vi "Copy Builds NI VeriStand dir.vi"(8 "error in (no error)":errorcluster, 9 "Custom Device Name":string="TimingDRV", 10 "VS Common Directory":string="Timing and Sync", 11 "CD Build Tools in":refnum<class "Project Build Tools.lvclass">) -> (0 "error out":errorcluster, 3 "CD Build Tools out":refnum<class "Project Build Tools.lvclass">)   [LabVIEW 2019, in "Project Build Tools.lvclass"]
doc: "This VI is called after each run of a build specification. The VI will copy the generated LLB (Engine or System Explorer) into the VeriStand Custom Device folder (...\\Documents\\National Instruments\\NI VeriStand 2013...)."
uses:
  Project Build Tools.lvclass
  <vilib>/Utility/sysdir.llb/System Directory Type.ctl
  Project Build Tools.lvclass/Project Build Tools.ctl
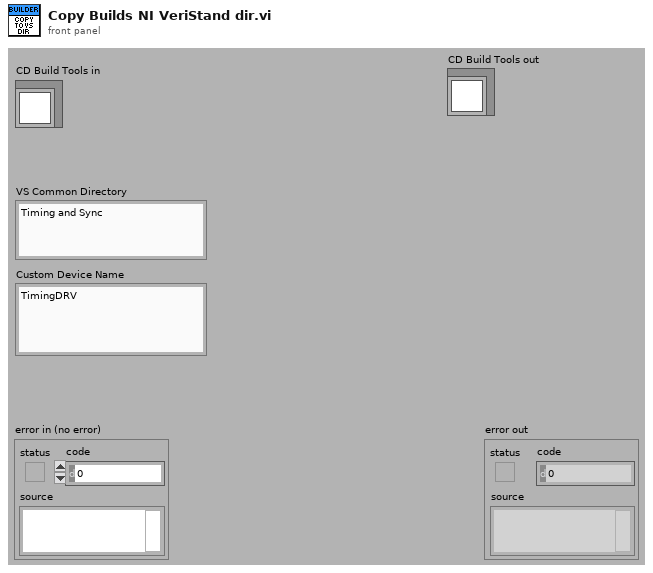
[diagram p1: front panel]
types:
  T1 = typedef "System Directory Type.ctl" = i32
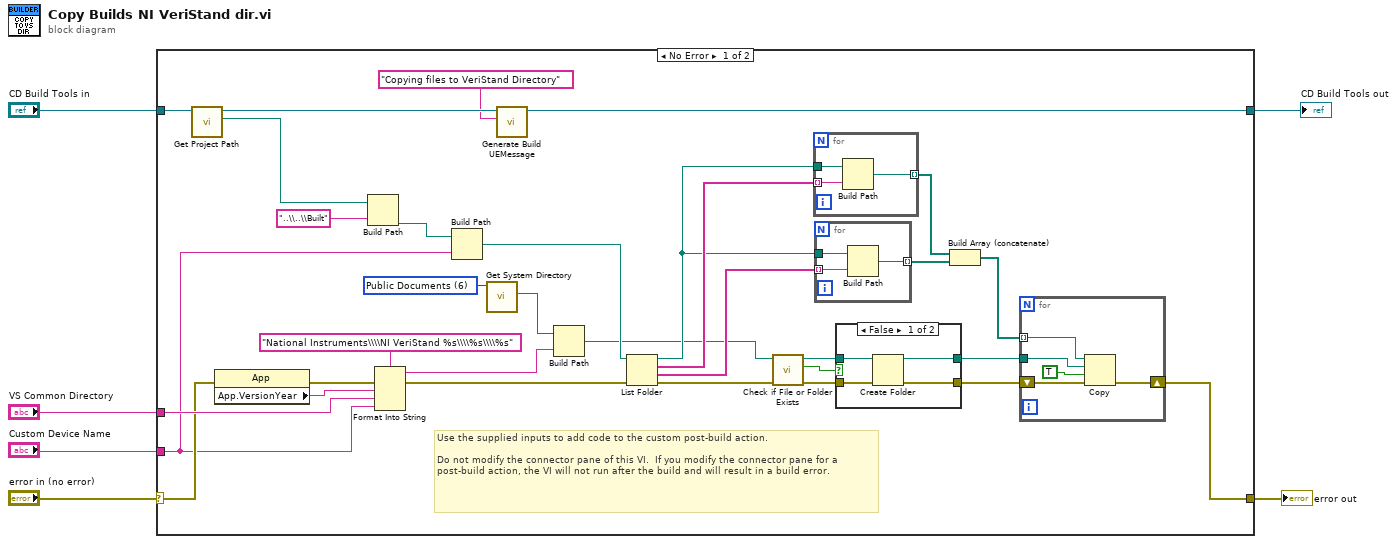
[diagram p0: block diagram]
diagram:
  n1 = case shown="No Error" "error in (no error)" {
    selector: "error in (no error)" -> [w17 w57]
    tunnel: [w20 w57] -> w5
    tunnel: "VS Common Directory" -> [w18 _]
    tunnel: "Custom Device Name" -> [w15 _]
    tunnel: "CD Build Tools in" -> [w11 w56]
    tunnel: [w7 w56] -> w1
    frame No Error {
      w24 = T1 6 items=["User Home"=0, "User Desktop"=1, "User Documents"=2, "User Application Data"=3, "User Preferences"=4, "User Temporary"=5, "Public Documents"=6, "Public Application Data"=7, "Public Preferences"=8, "Public Cache"=13, "System Core Libraries"=9, "System Installed Libraries"=10, "Application Files"=11, "Boot Volume Root"=12] ("system directory type")
      # "Use the supplied inputs to add code to the custom post-build action.\n\nDo not modify the connector pane of this VI.  If you modify the connector pane for a post-build action, the VI will not run after the build and will result in a build error."
      n2 = call "Get Project Path.vi"("CD Build Tools in"=w11) -> ("Project Path"=w10:path, "CD Build Tools out"=w9:refnum<class "Project Build Tools.lvclass">)  [unwired: 9 in]
      n3 = property class="App"(error in=w17) -> (error out=w23:errorcluster, "App.VersionYear"=w22:string)  [unwired: 1 in, 1 out]
      n4 = Build Path(base path=w10, name or relative path="..\\..\\Built") -> (appended path=w27:path)
      n5 = Format Into String(format string="National Instruments\\\\NI VeriStand %s\\\\%s\\\\%s" ("name or relative path"), error in=w23, w22, w18, w15) -> (resulting string=w26:string, error out=w16:errorcluster)  [unwired: 1 in]
      n6 = Build Path(base path=w27, name or relative path=w15) -> (appended path=w29:path)
      n7 = call <vilib>:"Get System Directory.vi"("system directory type"=w24) -> ("system directory"=w25:path)  [unwired: 10 in]
      n8 = call "Generate Build UEMessage.vi"("Message"="Copying files to VeriStand Directory" ("event data"), "Project Build Tools in"=w9) -> ("Project Build Tools out"=w7:refnum<class "Project Build Tools.lvclass">)  [unwired: 8 in, 1 out]
      n9 = Build Path(base path=w25, name or relative path=w26) -> (appended path=w19:path)
      n10 = List Folder(path=w29, error in=w16) -> (path out=w31:path, filenames=w38:string[], folder names=w32:string[], error out=w28:errorcluster)  [unwired: 2 in]
      n11 = call <vilib>:"Check if File or Folder Exists.vi"("error in (no error)"=w28, "path"=w19) -> ("error out"=w33:errorcluster, "file or folder exists?"=w35:bool, "dup path"=w34:path)  [unwired: 7 in]
      n12 = for {
        tunnel: w38 -> [w54] mode=indexing
        tunnel: w31 -> [w55]
        tunnel: [w53] -> w37 mode=indexing
        n13 = Build Path(base path=w55, name or relative path=w54) -> (appended path=w53:path)
      }
      n14 = for {
        tunnel: w32 -> [w51] mode=indexing
        tunnel: w31 -> [w52]
        tunnel: [w50] -> w30 mode=indexing
        n15 = Build Path(base path=w52, name or relative path=w51) -> (appended path=w50:path)
      }
      n16 = case shown="False" w35 {
        tunnel: w34 -> [w42 w44]
        tunnel: w33 -> [w41 w43]
        tunnel: [w40 w44] -> w13
        tunnel: [w39 w43] -> w12
        frame False {
          n17 = Create Folder(path (use dialog)=w42, error in=w41) -> (created path=w40:path, error out=w39:errorcluster)  [unwired: 1 in, 1 out]
        }
        frame True {
        }
      }
      n18 = Build Array (concatenate)(w37, w30) -> (w36:path[])
      n19 = for {
        tunnel: w36 -> [w46] mode=indexing
        shift-right: [w47] -> w20
        shift-left: w12 -> [w48]
        tunnel: w13 -> [w45]
        n20 = Copy(8:w48, 9:TRUE ("overwrite (F)"), 10:w45, 11:w46) -> (0:w47:errorcluster)  [unwired: 1 in, 2 out]
      }
    }
    frame Error {
    }
  }
  "error out" <- w5
  "CD Build Tools out" <- w1
